vi "launch_test_2.vi"(8 "error in (no error)":errorcluster, 9 "Message Queues in":T2, 11 "test mode":T1(ring)) -> (0 "error out":errorcluster)   [LabVIEW 2015]
uses:
  support/Message Queue/All Message Queues.ctl
  support/Message Queue/Message Cluster.ctl
  support/Message Queue/Enqueue Message (Array).vi
  support/Message Queue/Message Queue.lvlib
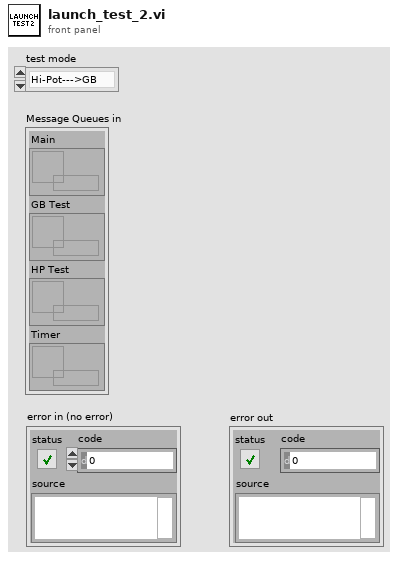
[diagram p1: front panel]
types:
  T1 = enum16{"Hi-Pot--->GB", "GB--->Hi-Pot", "Hi-Pot only", "GB only"}
  T2 = typedef "Message Queue.lvlib/All Message Queues.ctl" = cluster{"Main":refnum<queue>, "GB Test":refnum<queue>, "HP Test":refnum<queue>, "Timer":refnum<queue>}
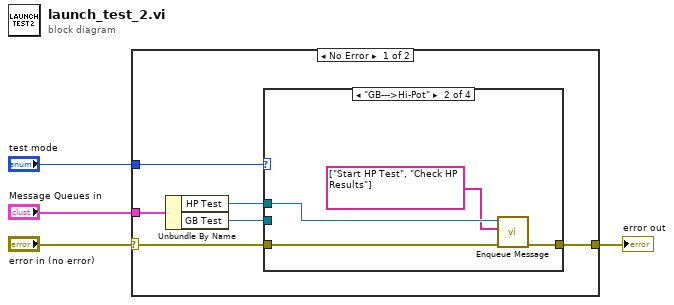
[diagram p0: block diagram]
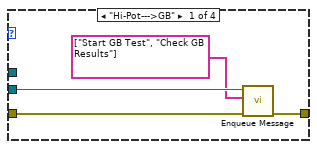
[diagram p2: hidden frame]
diagram:
  n1 = case shown="No Error" "error in (no error)" {
    selector: "error in (no error)" -> [w6 w21]
    tunnel: "Message Queues in" -> [w8 _]
    tunnel: "test mode" -> [w7 _]
    tunnel: [w5 w21] -> w1
    frame No Error {
      n2 = Unbundle By Name(w8) -> ("HP Test"=w9:refnum<queue>, "GB Test"=w10:refnum<queue>)
      n3 = case shown="\"GB--->Hi-Pot\"" w7 {
        tunnel: w9 -> [_ w18 _ _]
        tunnel: w10 -> [w14 _ _ _]
        tunnel: w6 -> [w12 w16 w19 w20]
        tunnel: [w11 w15 w19 w20] -> w5
        frame "Hi-Pot--->GB" {
          n4 = call-poly "Enqueue Message.vi"("error in (no error)"=w12, "Message Array"=string[] ["Start GB Test", "Check GB Results"], "Message Queue"=w14) -> ("error out"=w11:errorcluster)  [unwired: 7 in, 1 out]
        }
        frame "GB--->Hi-Pot" {
          n5 = call-poly "Enqueue Message.vi"("error in (no error)"=w16, "Message Array"=string[] ["Start HP Test", "Check HP Results"], "Message Queue"=w18) -> ("error out"=w15:errorcluster)  [unwired: 7 in, 1 out]
        }
        frame "GB only" {
        }
        frame "Hi-Pot only" {
        }
      }
    }
    frame Error {
    }
  }
  "error out" <- w1
